vi "Read.vi"(7 "timeout (100ms)":i32=100, 8 "error in (no error)":errorcluster, 9 "Interlock in":bool, 11 "Interlock Deny in":refnum<class "IL I32 Seize.lvclass">) -> (0 "error out":errorcluster, 1 "Interlock out":bool, 2 "Data out":variant, 3 "Interlock Deny out":refnum<class "IL I32 Seize.lvclass">, 4 "IL Action":refnum<class "IL Action.lvclass">[](array[class]))   [LabVIEW 2015, in "Interlocks.lvlib" / "IL I32 Seize.lvclass"]
uses:
  IL I32 Seize.lvclass
  IL Action/IL Action.lvclass
  IL I32 Seize.lvclass/IL I32 Seize.ctl
  Interlock/State Enum.ctl
  Interlock/Interlock.lvclass/Interlock.ctl
  Interlock/Interlock.lvclass
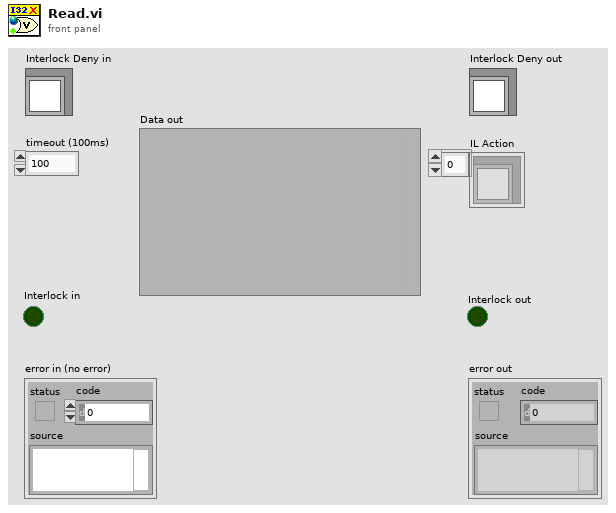
[diagram p1: front panel]
types:
  T1 = typedef "Interlocks.lvlib/Interlock.lvclass/State Enum.ctl" = enum16{"Ok", "Interlock", "Out of Range", "Is ON", "Is OFF", "Error", "Denied", "Not Allowed", "Sample Allow", "Sample Deny"}
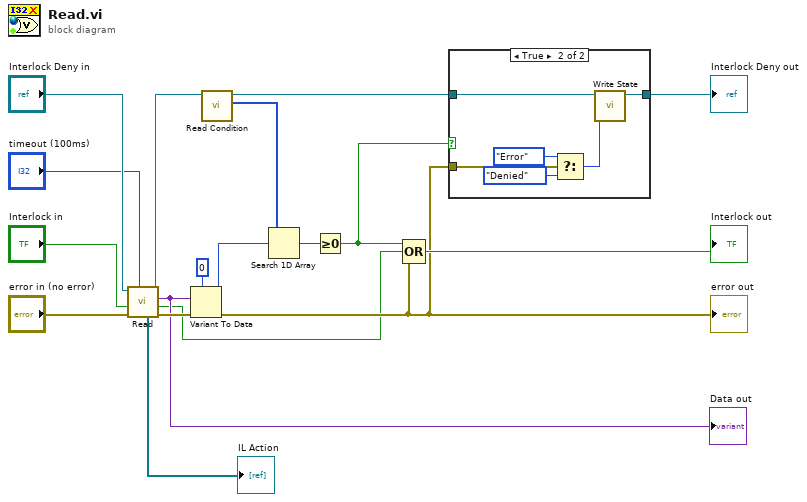
[diagram p0: block diagram]
diagram:
  n1 = call-parent "Read.vi"("timeout (100ms)"="timeout (100ms)", "error in (no error)"="error in (no error)", 9:"Interlock in"="Interlock in", 11:"Interlock in"="Interlock Deny in") -> ("error out"=w16:errorcluster, 1:"Interlock out"=w5:bool, "Data out"=w15:variant, 3:"Interlock out"=w12:refnum<class "IL I32 Seize.lvclass">, "IL Action"=→"IL Action":refnum<class "IL Action.lvclass">[])  [unwired: 3 in]
  "Data out" <- w15
  n2 = Variant To Data(error in=w16, type=0, Variant=w15) -> (data=w10:i32, error out=w6:errorcluster)
  "error out" <- w6
  n3 = call "Read Condition.vi"("Interlock Deny in"=w12) -> ("Deny"=w11:i32[], "Interlock Deny out"=w4:refnum<class "IL I32 Seize.lvclass">)  [unwired: 9 in]
  n4 = Search 1D Array(1D array=w11, element=w10) -> (index of element=w9:i32)  [unwired: 1 in]
  n5 = Greater Or Equal To 0?(x=w9) -> (x >= 0?=w7:bool)
  n6 = Compound Arithmetic op=OR(w7, w5, w6) -> (→"Interlock out":bool)
  n7 = case shown="True" w7 {
    tunnel: w6 -> [_ w25]
    tunnel: w4 -> [w19 w22]
    tunnel: [w19 w21] -> w3
    frame False {
    }
    frame True {
      n8 = Select(t=State_Enum."Error", s=w25, f=State_Enum."Denied" ("State")) -> (s? t:f=w20:T1)
      n9 = call "Write State.vi"("State"=w20, "Interlock in"=w22) -> ("Interlock out"=w21:refnum<class "IL I32 Seize.lvclass">)  [unwired: 9 in]
    }
  }
  "Interlock Deny out" <- w3
